vi "Remove Deadzone.vi"(10 "Deadzone (0.025)":dbl=0.025 format="%#_13g", 11 "Value":dbl) -> (2 "Sign":i32, 3 "Abs Value":dbl)   [LabVIEW 2019, in "User Interface.lvlib"]
doc: "Calculate the true value of the input by removing the deadzone. If the value is within the deadzone, the output is 0. Assumes input will be in range -/+ (1.0 + deadzone)."
uses:
  User Interface.lvlib
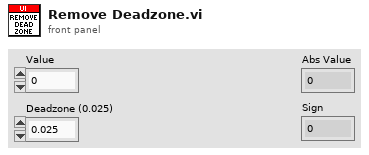
[diagram p1: front panel]
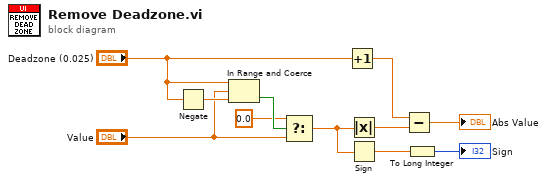
[diagram p0: block diagram]
diagram:
  n1 = Negate(x="Deadzone (0.025)") -> (-x=w11:dbl)
  n2 = In Range and Coerce(upper limit="Deadzone (0.025)", x="Value", lower limit=w11) -> (In Range?=w10:bool)  [unwired: 1 out]
  n3 = Select(t=0.0, s=w10, f="Value") -> (s? t:f=w7:dbl)
  n4 = Increment(x="Deadzone (0.025)") -> (x+1=w3:dbl)
  n5 = Absolute Value(x=w7) -> (abs(x)=w8:dbl)
  n6 = Sign(1:w7) -> (0:w6:dbl)
  n7 = Subtract(x=w3, y=w8) -> (x-y=→"Abs Value":dbl)
  n8 = To Long Integer(number=w6) -> (32bit integer=→"Sign":i32)
